vi "Init.vi"(8 "error in (no error)":errorcluster, 10 "Instrument String":variant, 11 "FPGA:R-Series in":refnum<class "R-Series.lvclass">) -> (0 "error out":errorcluster, 2 "Found?":bool=TRUE, 3 "FPGA:R-Series out":refnum<class "R-Series.lvclass">)   [LabVIEW 2025, in "FPGA.lvlib" / "R-Series.lvclass"]
uses:
  R-Series.lvclass
  C:/Working copy/tss/Plugin/Engines/FPGA/FPGA Instrument/FPGA Instrument.lvclass
  FPGA configuration/FPGA configuration.lvclass
  C:/Users/Public/Documents/Sandia National Labs/TSS Plugin/Abstract Engine.lvlibp/Instrument configuration/Instrument configuration.lvclass
  R-Series.lvclass/R-Series.ctl
  Users/Public/Documents/Sandia National Labs/TSS Plugin/Abstract Engine.lvlibp/Instrument configuration/Read Instrument Setting.vi
  Users/Public/Documents/Sandia National Labs/TSS Plugin/CEF.lvlibp/serializable configuration/CEF_serializable configuration.lvclass
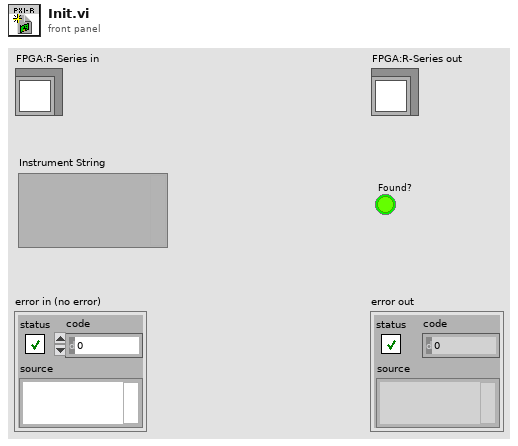
[diagram p1: front panel]
types:
  T1 = typedef "Abstract Engine.lvlibp/Instrument configuration.lvclass/Default Instrument.ctl" = cluster{"Type":string, "Address":string, "SW Alias":string, "Description":string, "Enabled":bool}
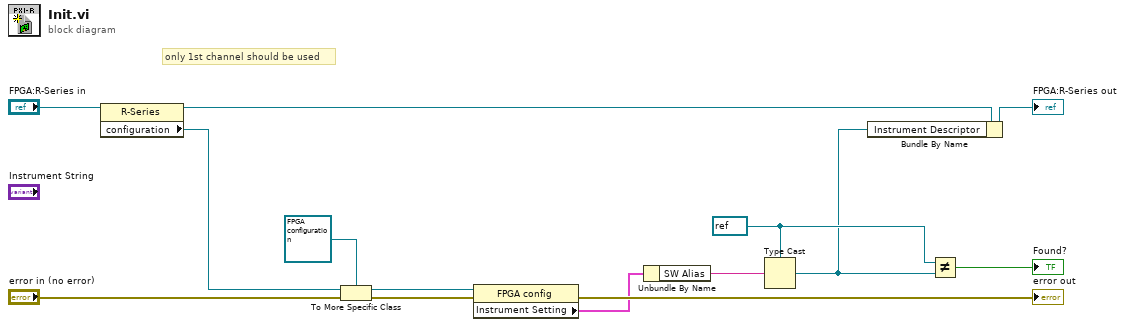
[diagram p0: block diagram]
diagram:
  w3 = refnum<k15> refnum ("instrument handle out")
  # "only 1st channel should be used"
  n1 = property class="R-Series"(reference="FPGA:R-Series in") -> (reference out=w11:refnum<class "R-Series.lvclass">, "configuration"=w9:refnum<class "CEF_serializable configuration.lvclass">)  [unwired: 1 in, 1 out]
  n2 = To More Specific Class(target class=refnum<class "FPGA configuration.lvclass"> refnum ("DMM.lvlib:DMM configuration.lvclass"), reference=w9, error in="error in (no error)") -> (specific class reference=w10:refnum<class "FPGA configuration.lvclass">, error out=w7:errorcluster)
  n3 = property class="FPGA config"(reference=w10, error in=w7) -> (error out=→"error out":errorcluster, "Instrument Setting"=w1:T1)  [unwired: 1 out]
  n4 = Unbundle By Name(w1) -> ("SW Alias"=w4:string)
  n5 = Type Cast(type=w3, x=w4) -> (*(type *) &x=w2:refnum<k15>)
  n6 = Bundle By Name(cluster=w11, "Instrument Descriptor"=w2) -> (→"FPGA:R-Series out":refnum<class "R-Series.lvclass">)
  n7 = Not Equal?(x=w3, y=w2) -> (x != y?=→"Found?":bool)
